vi "Python_Ref.vi"(0 "session in":refnum<k35>, 7 "Action":enum16{"Set Ref", "Get Ref"}(ring), 11 "Error In":errorcluster) -> (4 "session out":refnum<k35>, 15 "Error Out":errorcluster)   [LabVIEW 2023]
doc: "This VI gets or sets the GEA2 reference."
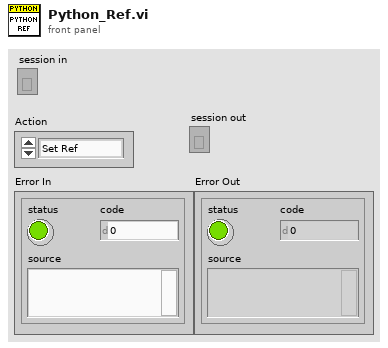
[diagram p1: front panel]
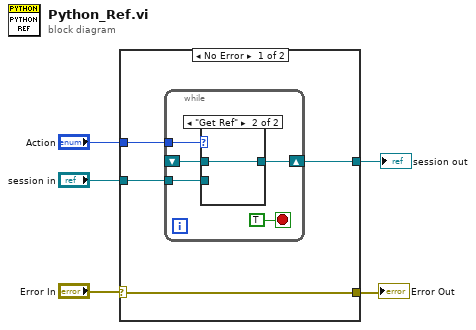
[diagram p0: block diagram]
diagram:
  n1 = case shown="No Error" "Error In" {
    selector: "Error In" -> [w6 w17]
    tunnel: "Action" -> [w9 _]
    tunnel: "session in" -> [w8 _]
    tunnel: [w7 _] -> w1
    tunnel: [w6 w17] -> w3
    frame No Error {
      n2 = while {
        tunnel: w9 -> [w13]
        tunnel: w8 -> [w12]
        shift-right: [w11] -> w7
        shift-left: _ -> [w10]
        stop <- TRUE stop-if-true
        n3 = case shown="\"Get Ref\"" w13 {
          tunnel: w12 -> [w15 _]
          tunnel: [w15 w16] -> w11
          tunnel: w10 -> [_ w16]
          frame "Set Ref" {
          }
          frame "Get Ref" {
          }
        }
      }
    }
    frame Error {
    }
  }
  "Error Out" <- w3
  "session out" <- w1
